vi "_Parse Named Range to Json.vi"(8 "error in (no error)":errorcluster, 10 "Named Range":string, 11 ".NET Refnum in":refnum<k24>) -> (0 "error out":errorcluster, 3 "Array":string[](array[string]))   [LabVIEW 2024, in "Config from EXCEL.lvclass"]
uses:
  Config from EXCEL.lvclass
  Config from EXCEL.lvclass/Config from EXCEL.ctl
  Open-Xml-LabVIEW/Source/Open Xml.lvlib
  D:/git/Open-Xml-LabVIEW/Source/DocumentFormat.OpenXml.dll
  Open-Xml-LabVIEW/Source/DocumentFormat.OpenXml.dll
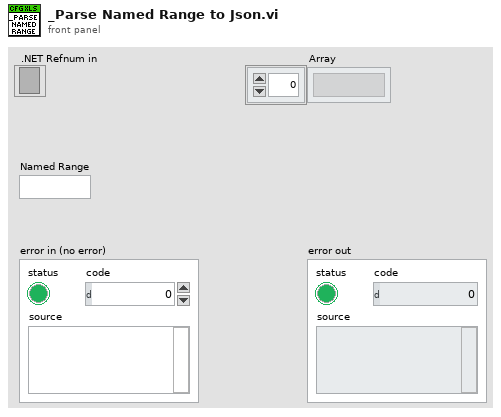
[diagram p1: front panel]
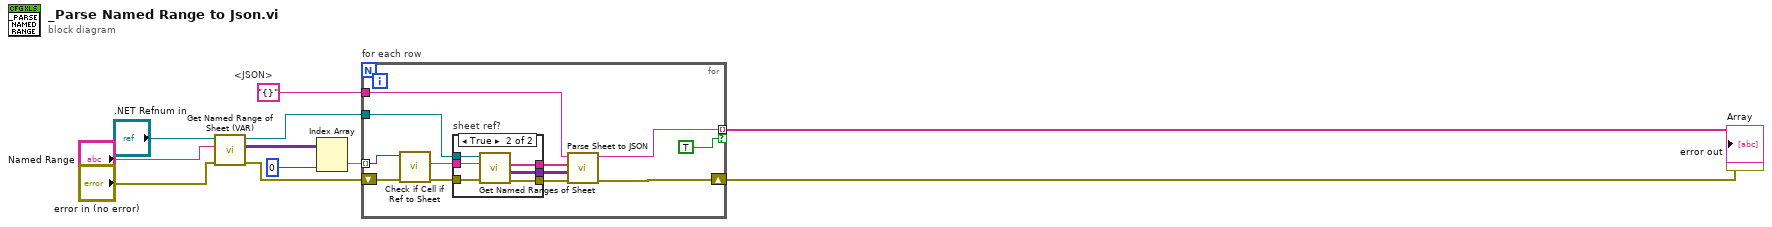
[diagram p0: block diagram]
diagram:
  w11 = "{}"  # <JSON>
  n1 = call "Get Named Range of Sheet (VAR).vi"("error in"="error in (no error)", "Named Range Identifier"="Named Range", "SpreadsheetDocument"=".NET Refnum in") -> ("error out"=w8:errorcluster, "Cells"=w4:variant[][], "SpreadsheetDocument out"=w7:refnum<k24>)  [unwired: 6 in]
  n2 = Index Array(array=w4, index (col)=0) -> (element=w5:variant[])  [unwired: 1 in]
  n3 = for "for each row" {
    tunnel: w5 -> [w19] mode=indexing
    tunnel: w7 -> [w20]
    shift-right: [w21] -> w9
    shift-left: w8 -> [w22]
    tunnel: [w18] -> w10 mode=indexing if=TRUE
    tunnel: w11 -> [w16]
    n4 = call "Check if Cell if Ref to Sheet.vi"("Value"=w19) -> ("Sheet Name"=w17:string)  [unwired: 9 in, 1 out]
    n5 = case "sheet ref?" shown="True" {
      selector: _ -> [_ _]
      tunnel: w22 -> [_ w28]
      tunnel: w20 -> [_ w27]
      tunnel: w17 -> [_ w26]
      tunnel: [_ w25] -> w15
      tunnel: [_ w24] -> w14
      tunnel: [_ w23] -> w13
      frame False {
      }
      frame True {
        n6 = call "Get Named Ranges of Sheet.vi"("error in"=w28, "Sheet Name"=w26, "SpreadsheetDocument"=w27) -> ("error out"=w25:errorcluster, "Cells"=w23:variant[][][], "Range Names"=w24:string[])  [unwired: 5 in, 1 out]
      }
    }
    n7 = call "Parse Sheet to JSON.vi"("error in"=w15, "Cells"=w13, "Named Ranges"=w14, "<JSON> in"=w16) -> ("error out"=w21:errorcluster, "<JSON> out"=w18:string)  [unwired: 6 in]
  }
  "Array" <- w10
  "error out" <- w9
